vi "TimeKeeping.vi"(7 "dt desired (ms)":u32=200, 8 "start tick":u32, 11 "Prev Loop Status":bool) -> (0 "time since start (s)":dbl, 3 "Current Loop Status":bool)   [LabVIEW 2025]
doc: "For conciseness. Flashes loop status as visual \nindicator for program function, stalls program\nloop execution by dt desired to maintain fixed \nsample time. Tracks time since start. Will only \nattempt to run at interval dt, server update \ncapped at 150ms dt.\n\nINPUTS:\n 1. Prev loop status -- bool\n 2. Clock at program init. -- int\n 3. Desired sample time -- int\n\nOUTPUTS:\n 1. Current loop status (inverted prev loop \n status) -- bool\n 2. Time since program start -- floating point\n DBL"
panel:
  # "Time Keeping\n\nFor conciseness. Flashes loop status as visual \nindicator for program function, stalls program\nloop execution by dt desired to maintain fixed \nsample time. Tracks time since start. Will only \nattempt to run at interval dt, server update \ncapped at 150ms dt.\n\nINPUTS:\n  1. Prev loop status -- bool\n  2. Clock at program init. -- int\n  3. Desired sample time -- int\n\nOUTPUTS:\n   1. Current loop status (inverted prev loop \n       status) -- bool\n   2. Time since program start -- floating point\n       DBL"
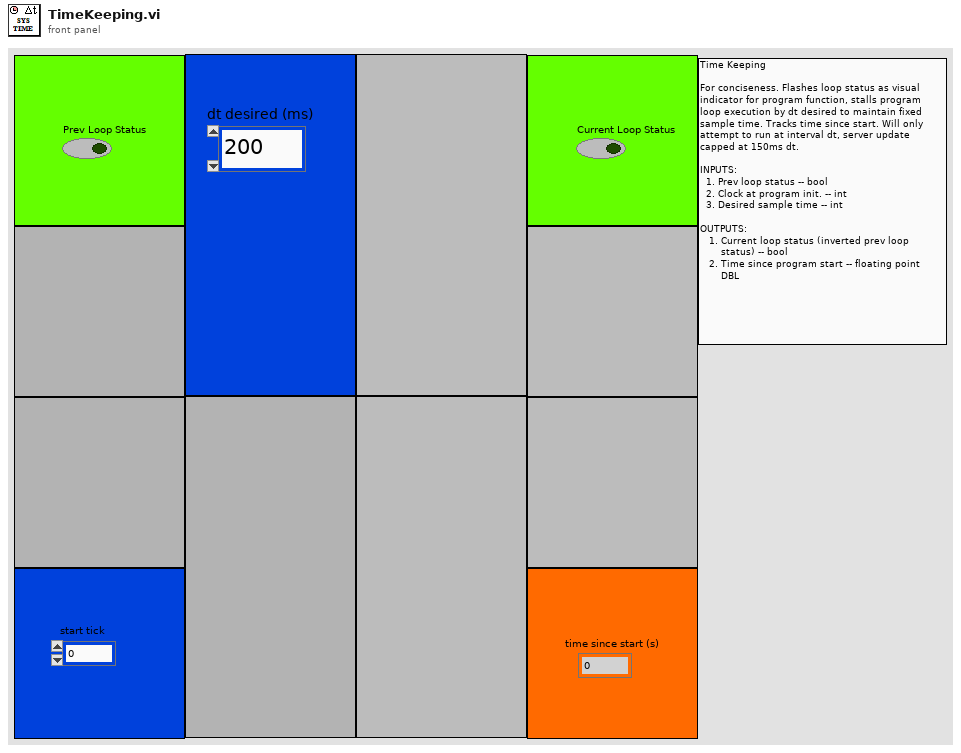
[diagram p1: front panel]
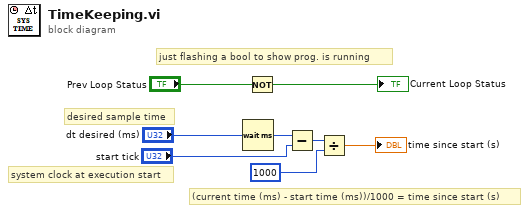
[diagram p0: block diagram]
diagram:
  # "just flashing a bool to show prog. is running"
  # "system clock at execution start"
  # "desired sample time"
  # "(current time (ms) - start time (ms))/1000 = time since start (s)"
  n1 = Wait (ms)(milliseconds to wait="dt desired (ms)") -> (millisecond timer value=w4:u32)
  n2 = Not(x="Prev Loop Status") -> (.not. x?=→"Current Loop Status":bool)
  n3 = Subtract(x=w4, y="start tick") -> (x-y=w1:u32)
  n4 = Divide(x=w1, y=u32 1000) -> (x/y=→"time since start (s)":dbl)
